vi "Create Element Hierarchy.vi"(6 "Name":string, 8 "error in (no error)":errorcluster, 9 "Parent":i32, 10 "Configs":map{i32, T1}(c390)) -> (0 "error out":errorcluster, 2 "Hierarchy":string[](array[string]))   [LabVIEW 2020, in "CDM-Config.lvlib" / "Config-Sqlite.lvclass"]
uses:
  Config-Sqlite.lvclass
  Config.ctl
  Meta Data.ctl
  CDM-Config.lvlib
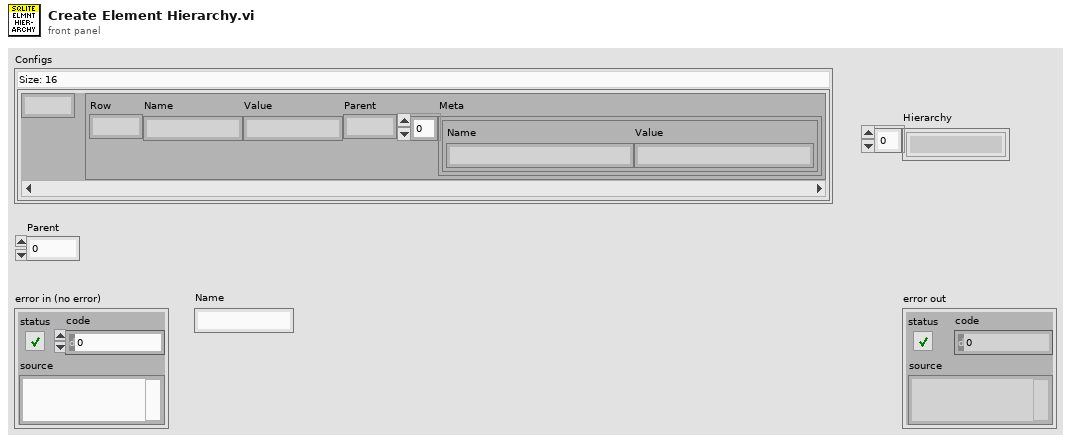
[diagram p1: front panel]
types:
  T1 = typedef "CDM-Config.lvlib/Config-Sqlite.lvclass/Config.ctl" = cluster{"Row":i32, "Name":string, "Value":string, "Parent":i32, "Meta":T2[]}
  T2 = typedef "CDM-Config.lvlib/Meta Data.ctl" = cluster{"Name":string, "Value":string}
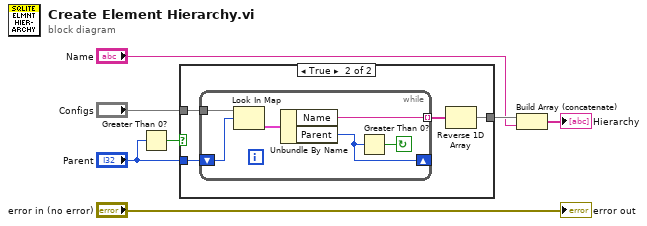
[diagram p0: block diagram]
diagram:
  n1 = Greater Than 0?(x="Parent") -> (x > 0?=w1:bool)
  n2 = case shown="True" w1 {
    tunnel: "Configs" -> [_ w11]
    tunnel: [_ w9] -> w5
    tunnel: "Parent" -> [_ w8]
    frame False {
    }
    frame True {
      n3 = while {
        tunnel: w11 -> [w17]
        shift-right: [w14] -> _
        shift-left: w8 -> [w16]
        tunnel: [w12] -> w10 mode=indexing
        stop <- w13 continue-if-true
        n4 = Look In Map(map=w17, key=w16) -> (value=w15:T1)  [unwired: 1 in, 1 out]
        n5 = Unbundle By Name(w15) -> ("Name"=w12:string, "Parent"=w14:i32)
        n6 = Greater Than 0?(x=w14) -> (x > 0?=w13:bool)
      }
      n7 = Reverse 1D Array(array=w10) -> (reversed array=w9:string[])
    }
  }
  n8 = Build Array (concatenate)(w5, "Name") -> (→"Hierarchy":string[])
  "error out" <- "error in (no error)"
